vi "ImageConstructer(MultilineBuffer).vi"(6 "Image Params":T1={"File Header"={"Start Position"=[], "StepWidth"=[0.05, 0.05], "Dimension"=[], "SpecLength"=10000}, "mzCali."=[0.0, 1.0, 0.0], "m/z_Array"=[0.0, 1.0, 0.0], "SampleRate"=0.0, "TrigDelay"=0.0, "file refnum"=refnum, "file path"=path "", "PeakOI"=[], "Binning"={"Enable"=FALSE, "BinType"=enum."ByScreen", "BinWidth"=0.5, "Maximum"=0.0, "Minimum"=0.0}} {"SampleRate" items=["50MS/s"=50000000.0, "100MS/s"=100000000.0, "125MS/s"=125000000.0, "200MS/s"=200000000.0, "250MS/s"=250000000.0, "500MS/s"=500000000.0, "1GS/s"=1000000000.0, "1.6GS/s"=1600000000.0, "2GS/s"=2000000000.0, "4GS/s"=4000000000.0]}, 7 "Image in":dbl[][][](array[numeric]), 8 "error in":errorcluster, 9 "AveCtr in":i32[](array[numeric]), 10 "ImageBuffer in":sgl[](array[numeric]), 11 "Y_img":i32) -> (0 "error out":errorcluster, 1 "AveCtr out":i32[](array[numeric]), 2 "ImageBuffer out":sgl[](array[numeric]), 3 "file refnum out":refnum<file>, 5 "Image out":dbl[][][](array[numeric]))   [LabVIEW 2014]
uses:
  ProcessMethods/BioMapConversion/BioMAPWriterCoreParams.ctl
  Files/BinaryHeader.ctl
  ControlDef/SampleRateSelector.ctl
  ProcessMethods/Binning/BinType.ctl
  <userlib>/Utility/ErrorLog_lib.lvlib
panel:
  out "size(s)":i32
  out "Array 2":i32[](array[numeric])
  out "Array":dbl[](array[numeric])
  out "AverageArray":sgl[](array[numeric])
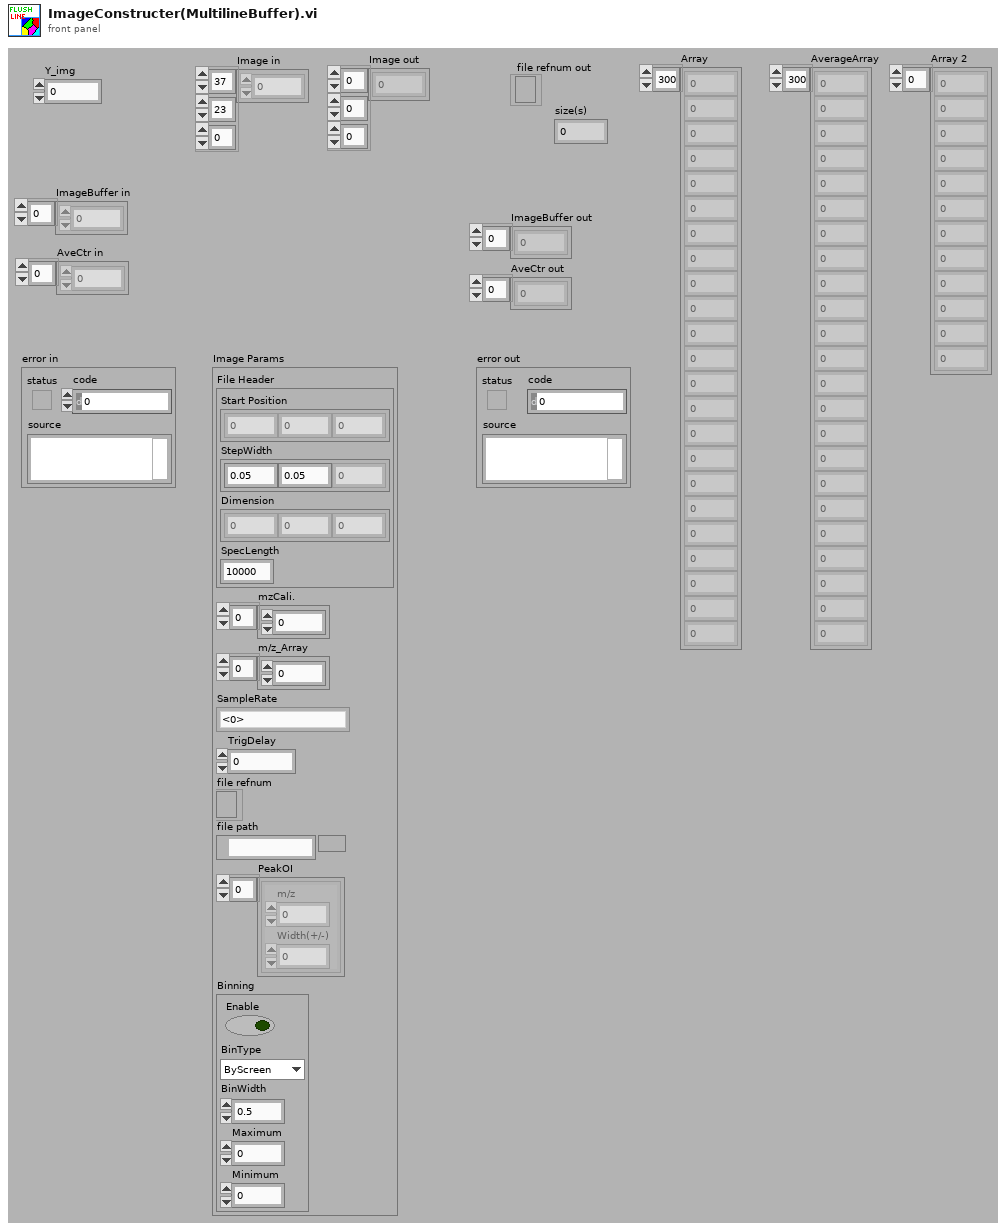
[diagram p1: front panel]
types:
  T1 = typedef "BioMAPWriterCoreParams.ctl" = cluster{"File Header":T2, "mzCali.":dbl[], "m/z_Array":dbl[], "SampleRate":T3, "TrigDelay":dbl, "file refnum":refnum<file>, "file path":path, "PeakOI":cluster{"m/z":dbl, "Width(+/-)":dbl}[], "Binning":cluster{"Enable":bool, "BinType":T4, "BinWidth":dbl, "Maximum":dbl, "Minimum":dbl}}
  T2 = typedef "BinaryHeader.ctl" = cluster{"Start Position":dbl[], "StepWidth":dbl[], "Dimension":i32[], "SpecLength":i32}
  T3 = typedef "SampleRateSelector.ctl" = dbl
  T4 = typedef "BinType.ctl" = enum16{"ByTime", "ByScreen", "ByMass", "ToUnitMass"}
  T5 = enum16{"big-endian, network order", "native, host order", "little-endian"}
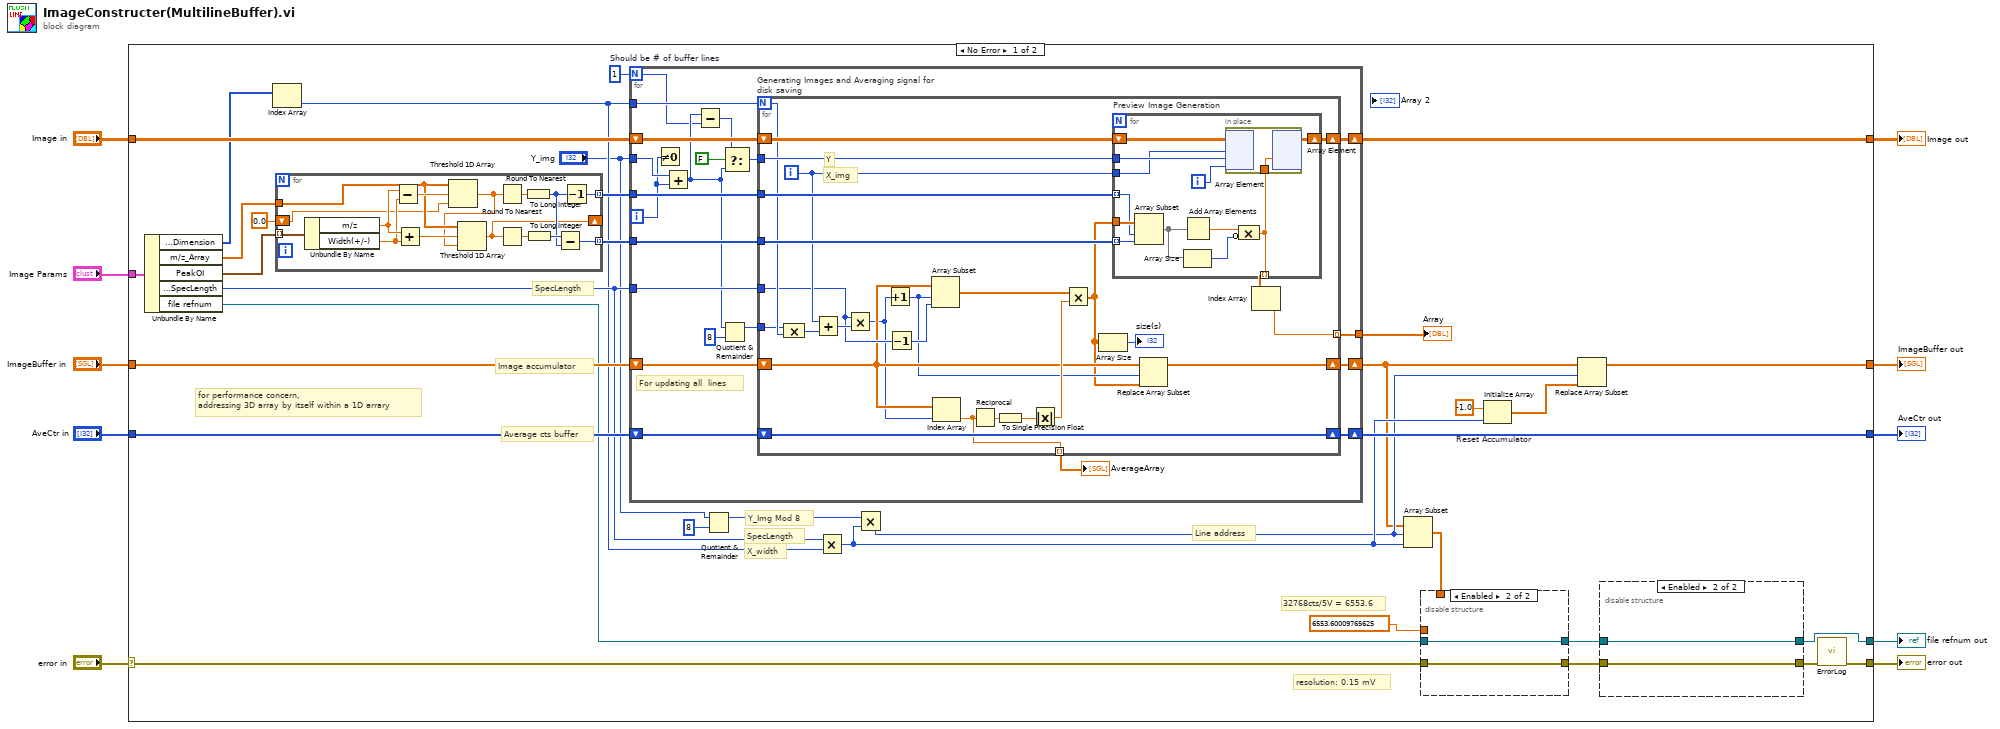
[diagram p0: block diagram]
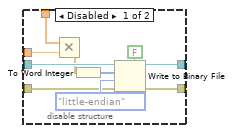
[diagram p2: hidden frame]
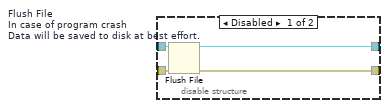
[diagram p3: hidden frame]
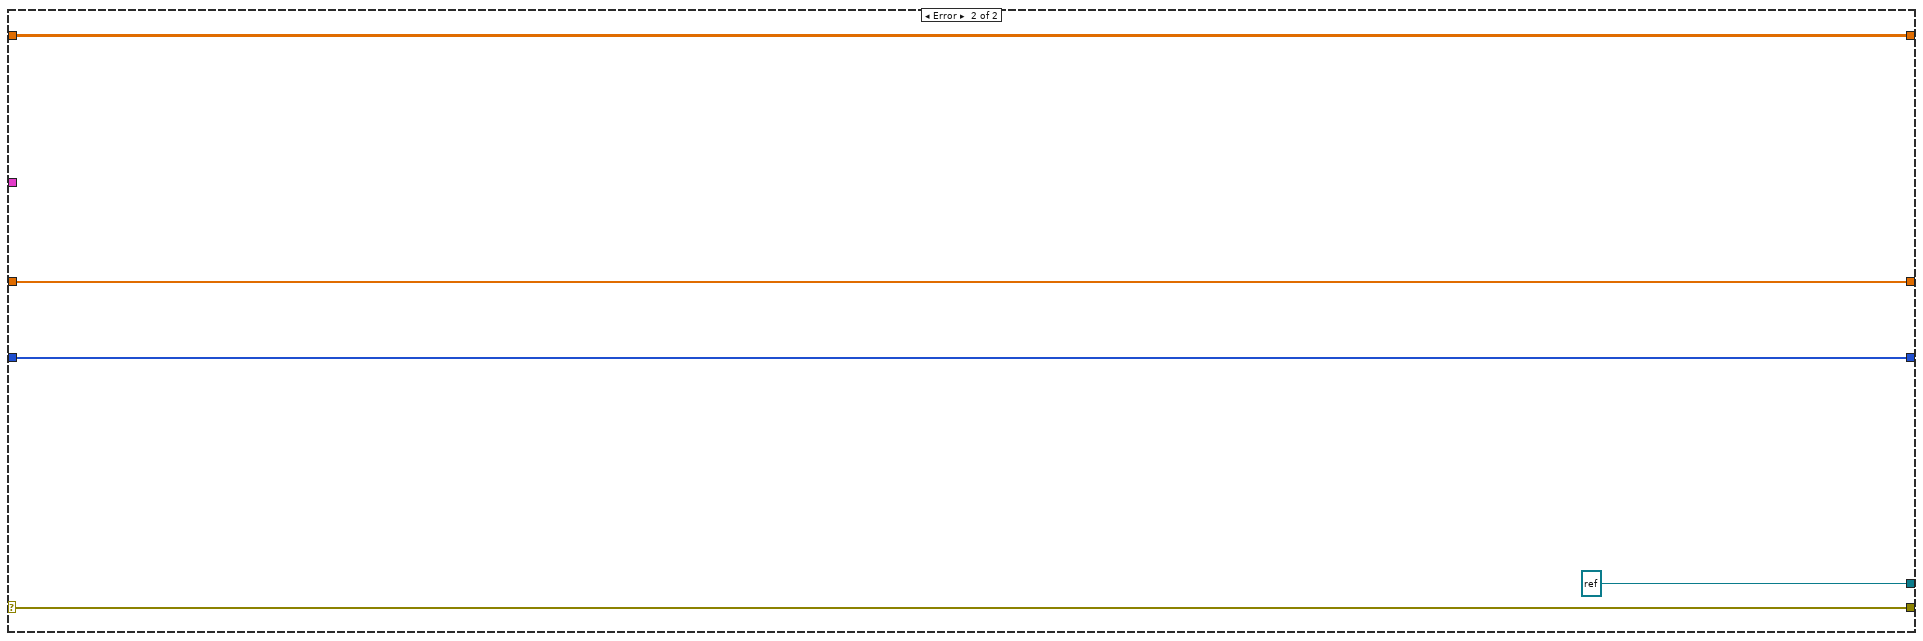
[diagram p4: hidden frame]
diagram:
  n1 = case shown="No Error" "error in" {
    selector: "error in" -> [w30 w142]
    tunnel: [w44 w140] -> w10
    tunnel: [w26 w142] -> w9
    tunnel: [w41 refnum<file> refnum ("file refnum")] -> w8
    tunnel: "Image in" -> [w43 w140]
    tunnel: "Image Params" -> [w39 _]
    tunnel: "ImageBuffer in" -> [w34 w139]
    tunnel: "AveCtr in" -> [w33 w138]
    tunnel: [w18 w139] -> w4
    tunnel: [w24 w138] -> w1
    frame No Error {
      w13 = 1  # Should be # of buffer lines
      # "resolution: 0.15 mV"
      # "32768cts/5V = 6553.6"
      # "for performance concern, \naddressing 3D array by itself within a 1D arrary"
      # "Line address"
      # "Y_Img Mod 8"
      # "SpecLength"
      # "X_width"
      # "Image accumulator"
      # "Average cts buffer"
      # "SpecLength"
      n2 = Unbundle By Name(w39) -> ("File Header.Dimension"=w42:i32[], "m/z_Array"=w38:dbl[], "PeakOI"=w37:cluster{"m/z":dbl, "Width(+/-)":dbl}[], "File Header.SpecLength"=w28:i32, "file refnum"=w32:refnum<file>)
      n3 = Index Array(array=w42) -> (element=w27:i32)  [unwired: 1 in]
      n4 = for "Preview Image Generation" {
        tunnel: w37 -> [w137] mode=indexing
        tunnel: w38 -> [w133]
        tunnel: [w126] -> w36 mode=indexing
        tunnel: [w127] -> w35 mode=indexing
        shift-right: [w124] -> _
        shift-left: 0.0 -> [w123]
        n5 = Unbundle By Name(w137) -> ("m/z"=w136:dbl, "Width(+/-)"=w135:dbl)
        n6 = Subtract(x=w136, y=w135) -> (x-y=w134:dbl)
        n7 = Add(x=w136, y=w135) -> (x+y=w132:dbl)
        n8 = Threshold 1D Array(1:w123, 2:w134, 3:w133) -> (0:w125:dbl)
        n9 = Threshold 1D Array(1:w125, 2:w132, 3:w133) -> (0:w124:dbl)
        n10 = Round To Nearest(number=w125) -> (nearest integer value=w130:dbl)
        n11 = Round To Nearest(number=w124) -> (nearest integer value=w131:dbl)
        n12 = To Long Integer(number=w130) -> (32bit integer=w128:i32)
        n13 = To Long Integer(number=w131) -> (32bit integer=w129:i32)
        n14 = Subtract(x=w129, y=w128) -> (x-y=w127:i32)
        n15 = Decrement(x=w128) -> (x-1=w126:i32)
      }
      n16 = for {
        N: w13 -> [w48]
        tunnel: w36 -> [w63]
        tunnel: w35 -> [w62]
        tunnel: w28 -> [w59]
        tunnel: w27 -> [w58]
        tunnel: "Y_img" -> [w54]
        shift-right: [w56] -> w14
        shift-left: w34 -> [w61]
        shift-right: [w57] -> w24
        shift-left: w33 -> [w60]
        shift-right: [w65] -> w44
        shift-left: w43 -> [w64]
        tunnel: [w45] -> w12
        i -> [w51]
        # "For updating all  lines"
        n17 = Not Equal To 0?(x=w51) -> ()  [unwired: 1 out]
        n18 = Add(x=w54, y=w51) -> (x+y=w50:i32)
        n19 = Subtract(x=w50, y=w48) -> (x-y=w49:i32)
        n20 = Quotient & Remainder(x=w50, y=8) -> (x-y*floor(x/y)=w52:i32)  [unwired: 1 out]
        n21 = Select(t=w49, s=FALSE, f=w50) -> (s? t:f=w47:i32)
        n22 = for "Generating Images and Averaging signal for disk saving" {
          N: w58 -> [w85]
          shift-right: [w91] -> w65
          shift-left: w64 -> [w90]
          tunnel: w62 -> [w88]
          tunnel: w63 -> [w89]
          tunnel: w47 -> [w86]
          shift-right: [w81] -> w56
          shift-left: w61 -> [w73]
          shift-right: [w82] -> w57
          shift-left: w60 -> [w82]
          tunnel: [w74] -> w55 mode=indexing
          tunnel: w59 -> [w78]
          tunnel: w52 -> [w75]
          tunnel: [w66] -> w45 mode=indexing
          i -> [w84]
          # "Y"
          # "X_img"
          n23 = Compound Arithmetic op=MULTIPLY(w75, w85) -> (w87:i32)
          n24 = Add(x=w84, y=w87) -> (x+y=w83:i32)
          n25 = Multiply(x=w78, y=w83) -> (x*y=w72:i32)
          n26 = Increment(x=w72) -> (x+1=w70:i32)
          n27 = Decrement(x=w78) -> (x-1=w71:i32)
          n28 = Array Subset(array=w73, index=w70, length=w71) -> (w77:sgl[])
          n29 = Index Array(array=w73, index=w72) -> (element=w74:sgl)
          n30 = Reciprocal(x=w74) -> (1/x=w80:sgl)
          n31 = To Single Precision Float(number=w80) -> (single precision float=w79:sgl)
          n32 = Absolute Value(x=w79) -> (abs(x)=w76:sgl)
          n33 = Multiply(x=w77, y=w76) -> (x*y=w69:sgl[])
          n34 = Array Size(array=w69) -> (size(s)=→"size(s)":i32)
          n35 = for "Preview Image Generation" {
            shift-right: [w101] -> w91
            shift-left: w90 -> [w103]
            tunnel: w69 -> [w102]
            tunnel: w84 -> [w93]
            tunnel: w88 -> [w96] mode=indexing
            tunnel: w89 -> [w97] mode=indexing
            tunnel: w86 -> [w95]
            tunnel: [w92] -> w67 mode=indexing
            i -> [w94]
            n36 = Array Subset(array=w102, index=w97, length=w96) -> (w98:sgl[])
            n37 = Array Size(array=w98) -> (size(s)=w99:i32)
            n38 = Add Array Elements(numeric array=w98) -> (sum=w100:sgl)
            n39 = Compound Arithmetic op=MULTIPLY(w100, invert w99) -> (w92:dbl)
            n40 = in-place {
              in-place-border: w92 -> [w104]
              n41 = in-place-array #1(w103, w93, w95, w94) -> ()  [unwired: 1 out]
              n42 = in-place-array #1(w104) -> (w101:dbl[][][])  [unwired: 3 out]
            }
          }
          n43 = Replace Array Subset(array=w73, new element=w69, index=w70) -> (w81:sgl[])
          n44 = Index Array(array=w67) -> (element=w66:dbl)  [unwired: 1 in]
        }
        "AverageArray" <- w55
      }
      "Array" <- w12
      n45 = Quotient & Remainder(x="Y_img", y=8) -> (x-y*floor(x/y)=w22:i32)  [unwired: 1 out]
      n46 = Multiply(x=w28, y=w27) -> (x*y=w19:i32)
      n47 = Multiply(x=w22, y=w19) -> (x*y=w16:i32)
      n48 = Array Subset(array=w14, index=w16, length=w19) -> (w15:sgl[])
      n49 = disable-structure shown="Enabled" {
        disable-tunnel: w32 -> [w114 w116]
        disable-tunnel: [w113 w116] -> w31
        disable-tunnel: [w110 w115] -> w29
        disable-tunnel: w30 -> [w109 w115]
        disable-tunnel: w15 -> [w108 _]
        disable-tunnel: sgl 6553.6 -> [w105 _]
        frame Disabled {
          n50 = Multiply(x=w108, y=w105) -> (x*y=w106:sgl[])
          n51 = To Word Integer(number=w106) -> (16bit integer=w107:i16[])
          n52 = Write to Binary File(file (use dialog)=w114, data=w107, error in=w109, 5:FALSE ("prepend array or string size? (T)"), 9:T5."little-endian" ("byte order (0:big-endian, network order)")) -> (refnum out=w113:refnum<file>, error out=w110:errorcluster)  [unwired: 1 in, 1 out]
        }
        frame Enabled {
        }
      }
      n53 = Initialize Array "Reset Accumulator"(sgl -1.0, w19) -> (w17:sgl[])
      n54 = Replace Array Subset(array=w14, new element=w17, index=w16) -> (w18:sgl[])
      n55 = disable-structure shown="Enabled" {
        disable-tunnel: w31 -> [w120 w122]
        disable-tunnel: [w119 w122] -> w41
        disable-tunnel: w29 -> [w118 w121]
        disable-tunnel: [w117 w121] -> w40
        frame Disabled {
          n56 = Flush File "Flush File\nIn case of program crash\nData will be saved to disk at best effort."(refnum=w120, error in=w118) -> (refnum out=w119:refnum<file>, error out=w117:errorcluster)
        }
        frame Enabled {
        }
      }
      n57 = call <userlib>:"ErrorLog.vi"("error in (no error)"=w40) -> ("error out"=w26:errorcluster)  [unwired: 10 in]
    }
    frame Error {
    }
  }
  "Image out" <- w10
  "error out" <- w9
  "file refnum out" <- w8
  "ImageBuffer out" <- w4
  "AveCtr out" <- w1
